vi "Update Item Status.vi"(8 "error in (no error)":errorcluster, 9 "Status":T1, 10 "Test Case":string, 11 "Icon Decorator In":refnum<class "Icon Decorator.lvclass">) -> (0 "error out":errorcluster, 3 "Icon Decorator Out":refnum<class "Icon Decorator.lvclass">)   [LabVIEW 2020, in "Icon Decorator.lvclass"]
doc: "Set the status as an integer property saved in the project item."
uses:
  Icon Decorator.lvclass
  Rewrite Project/Result/Status.ctl
  Icon Decorator.lvclass/Icon Decorator.ctl
  Rewrite Project/Result/Result.lvlib
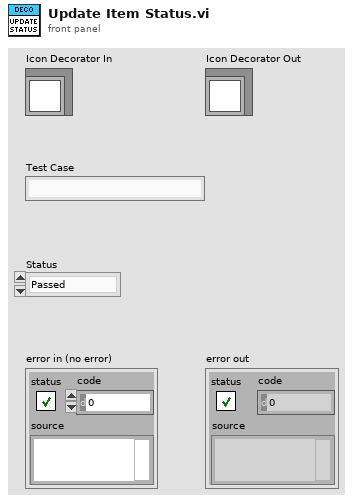
[diagram p1: front panel]
types:
  T1 = typedef "Result.lvlib/Status.ctl" = enum16{"Passed", "Failed", "Error", "Skipped", "Setup Error", "Broken", "Teardown Error"}
  T2 = typedef "ItemRef.ctl" = u64
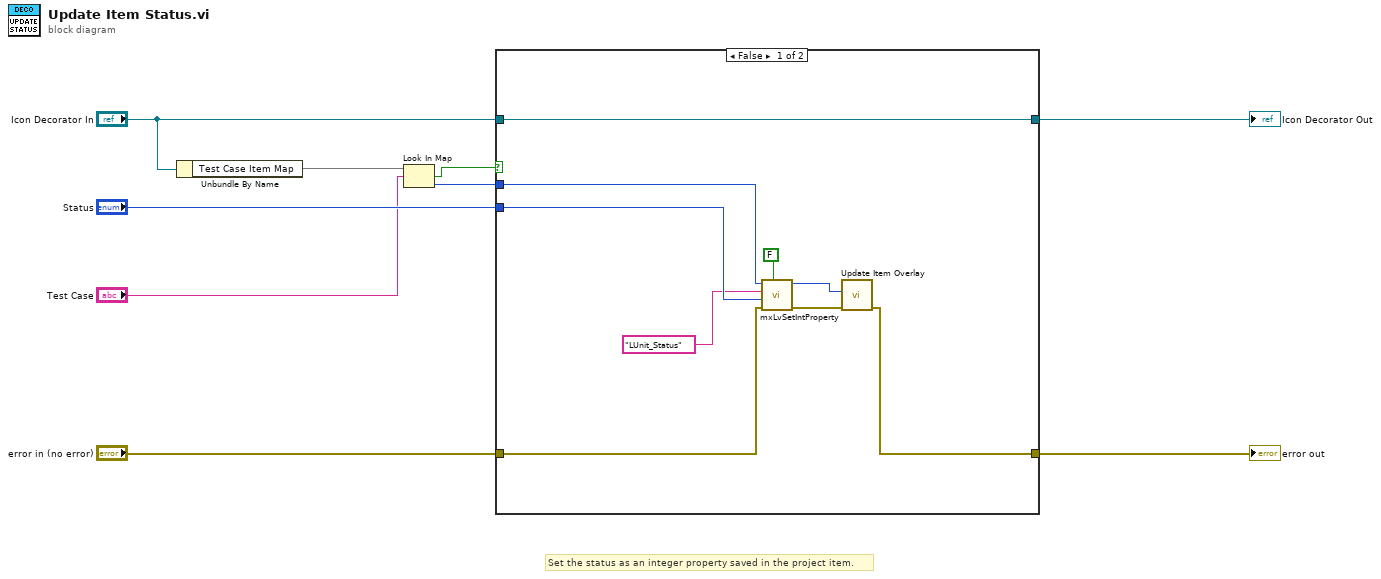
[diagram p0: block diagram]
diagram:
  # "Set the status as an integer property saved in the project item."
  n1 = Unbundle By Name("Icon Decorator In") -> ("Test Case Item Map"=w9:map{string, T2})
  n2 = Look In Map(map=w9, key="Test Case") -> (key not found?=w6:bool, value=w5:T2)  [unwired: 1 in]
  n3 = case shown="False" w6 {
    tunnel: "Icon Decorator In" -> [w18 w20]
    tunnel: [w18 w20] -> w3
    tunnel: [w16 w19] -> w4
    tunnel: "error in (no error)" -> [w17 w19]
    tunnel: w5 -> [w10 _]
    tunnel: "Status" -> [w15 _]
    frame False {
      n4 = call <resource>:"mxLvSetIntProperty.vi"("Persist Property? (T)"=FALSE, "error in"=w17, "Value (0)"=w15, "Tag"="LUnit_Status", "Item"=w10) -> ("error out"=w11:errorcluster, "Item"=w12:T2)  [unwired: 5 in]
      n5 = call "Update Item Overlay.vi"("error in (no error)"=w11, "Item"=w12) -> ("error out"=w16:errorcluster)  [unwired: 8 in, 1 out]
    }
    frame True {
    }
  }
  "error out" <- w4
  "Icon Decorator Out" <- w3
